vi "仪器地址读取.vi"(6 "error in (no error)":errorcluster caption="错误输入（无错误）") -> (0 "error out":errorcluster caption="错误输出", 3 "仪器地址":T1)   [LabVIEW 2021]
uses:
  <vilib>/Utility/config.llb/Read Key (String).vi
  <vilib>/Utility/config.llb/NI_LVConfig.lvlib
panel:
  out "拆分的路径":path
  out "添加的路径":path
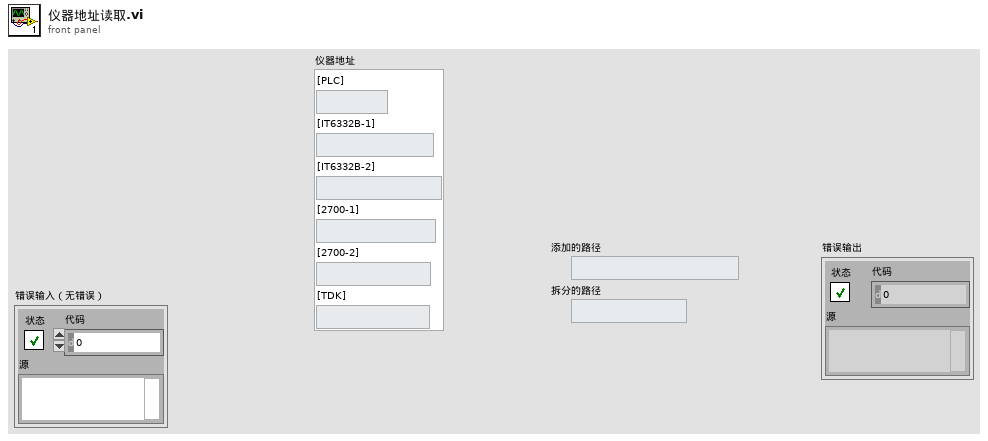
[diagram p1: front panel]
types:
  T1 = typedef "仪器地址输入.ctl" = cluster{"[PLC]":string, "[IT6332B-1]":string, "[IT6332B-2]":string, "[2700-1]":string, "[2700-2]":string, "[TDK]":string}
  T2 = typedef "NI_LVConfig.lvlib/Config Data RefNum.ctl" = refnum<k1>
  T3 = cluster{"[0]":string, "[1]":string, "[2]":string, "[3]":string, "[4]":string, "[5]":string}
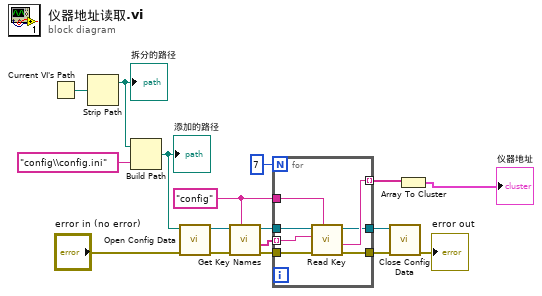
[diagram p0: block diagram]
diagram:
  w15 = "config" ("section")
  n1 = Current VI's Path() -> (path=w7:path)
  n2 = Strip Path(path=w7) -> (stripped path=w6:path)  [unwired: 1 out]
  "拆分的路径" <- w6
  n3 = Build Path(base path=w6, name or relative path="config\\config.ini") -> (appended path=w4:path)
  "添加的路径" <- w4
  n4 = call <vilib>:"Open Config Data.vi"("error in (no error)"="error in (no error)", "configuration file path"=w4) -> ("error out"=w12:errorcluster, "refnum"=w17:T2)  [unwired: 7 in, 1 out]
  n5 = call <vilib>:"Get Key Names.vi"("section"=w15, "error in (no error)"=w12, "refnum"=w17) -> ("error out"=w13:errorcluster, "key names"=w14:string[], "refnum out"=w16:T2)  [unwired: 5 in, 1 out]
  n6 = for {
    N: 7 -> [_]
    tunnel: w16 -> [w24]
    tunnel: w15 -> [w23]
    tunnel: w14 -> [w22] mode=indexing
    tunnel: w13 -> [w21]
    tunnel: [w20] -> w3 mode=indexing
    tunnel: [w19] -> w11
    tunnel: [w18] -> w10
    n7 = call-poly <vilib>:"Read Key.vi"("section"=w23, "error in (no error)"=w21, "key"=w22, "refnum"=w24) -> ("error out"=w19:errorcluster, "value"=w20:string, "refnum out"=w18:T2)  [unwired: 4 in, 1 out]
  }
  n8 = call <vilib>:"Close Config Data.vi"("error in (no error)"=w11, "refnum"=w10) -> ("error out"=→"error out":errorcluster)  [unwired: 8 in, 1 out]
  n9 = Array To Cluster(array=w3) -> (cluster=→"仪器地址":T3)
